vi "Simulation Acquired Data.vi"() -> ()   [LabVIEW 2013]
panel:
  in  "Data Queue":refnum<queue>
  in  "Skip Back Button":bool
  in  "FF Speed":dbl=2.0
  in  "Progress":dbl(slide)=0.002 scale=0.0..1435.0
  in  "Seek Forward Button":bool
  in  "Media Stop Button":bool
  in  "Play Button":bool
  in  "Tabs":enum32{"Config", "X", "Y", "Voltage"}(tab)
  in  "Reset Graphs":bool
  in  "TDMS File Name":string
  in  "TDMS Output Folder":path
  out "TDMS Path Result":path
  in  "View Data After?":bool
  out "X Position":cluster{"Y":dbl[], "Y":dbl[]}[](graph)
  out "Y Position":cluster{"Y":dbl[], "Y":dbl[]}[](graph)
  out "Tip Voltage":cluster{"Y":dbl[], "Y":dbl[]}[](graph)
  in  "Background Image":refnum<vi>
  in  "Inkscape File (.svg)":refnum<vi>
  in  "Run":refnum<vi>
  in  "Abort":refnum<vi>
  in  "Lithography Data":T1(array[cluster])
  # "Will be used for TDMS playback"
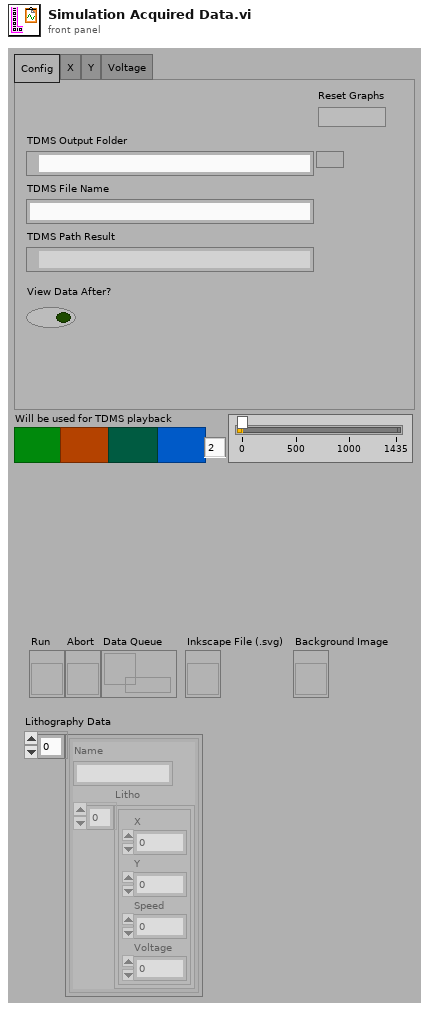
[diagram p1: front panel]
types:
  T1 = cluster{"Name":string, "Litho":cluster{"X":dbl, "Y":dbl, "Speed":dbl, "Voltage":dbl}[]}[]
  T2 = cluster{"X":dbl, "Y":dbl, "Speed":dbl, "Voltage":dbl}[]
  T3 = cluster{"X":dbl, "Y":dbl, "Speed":dbl, "Voltage":dbl}
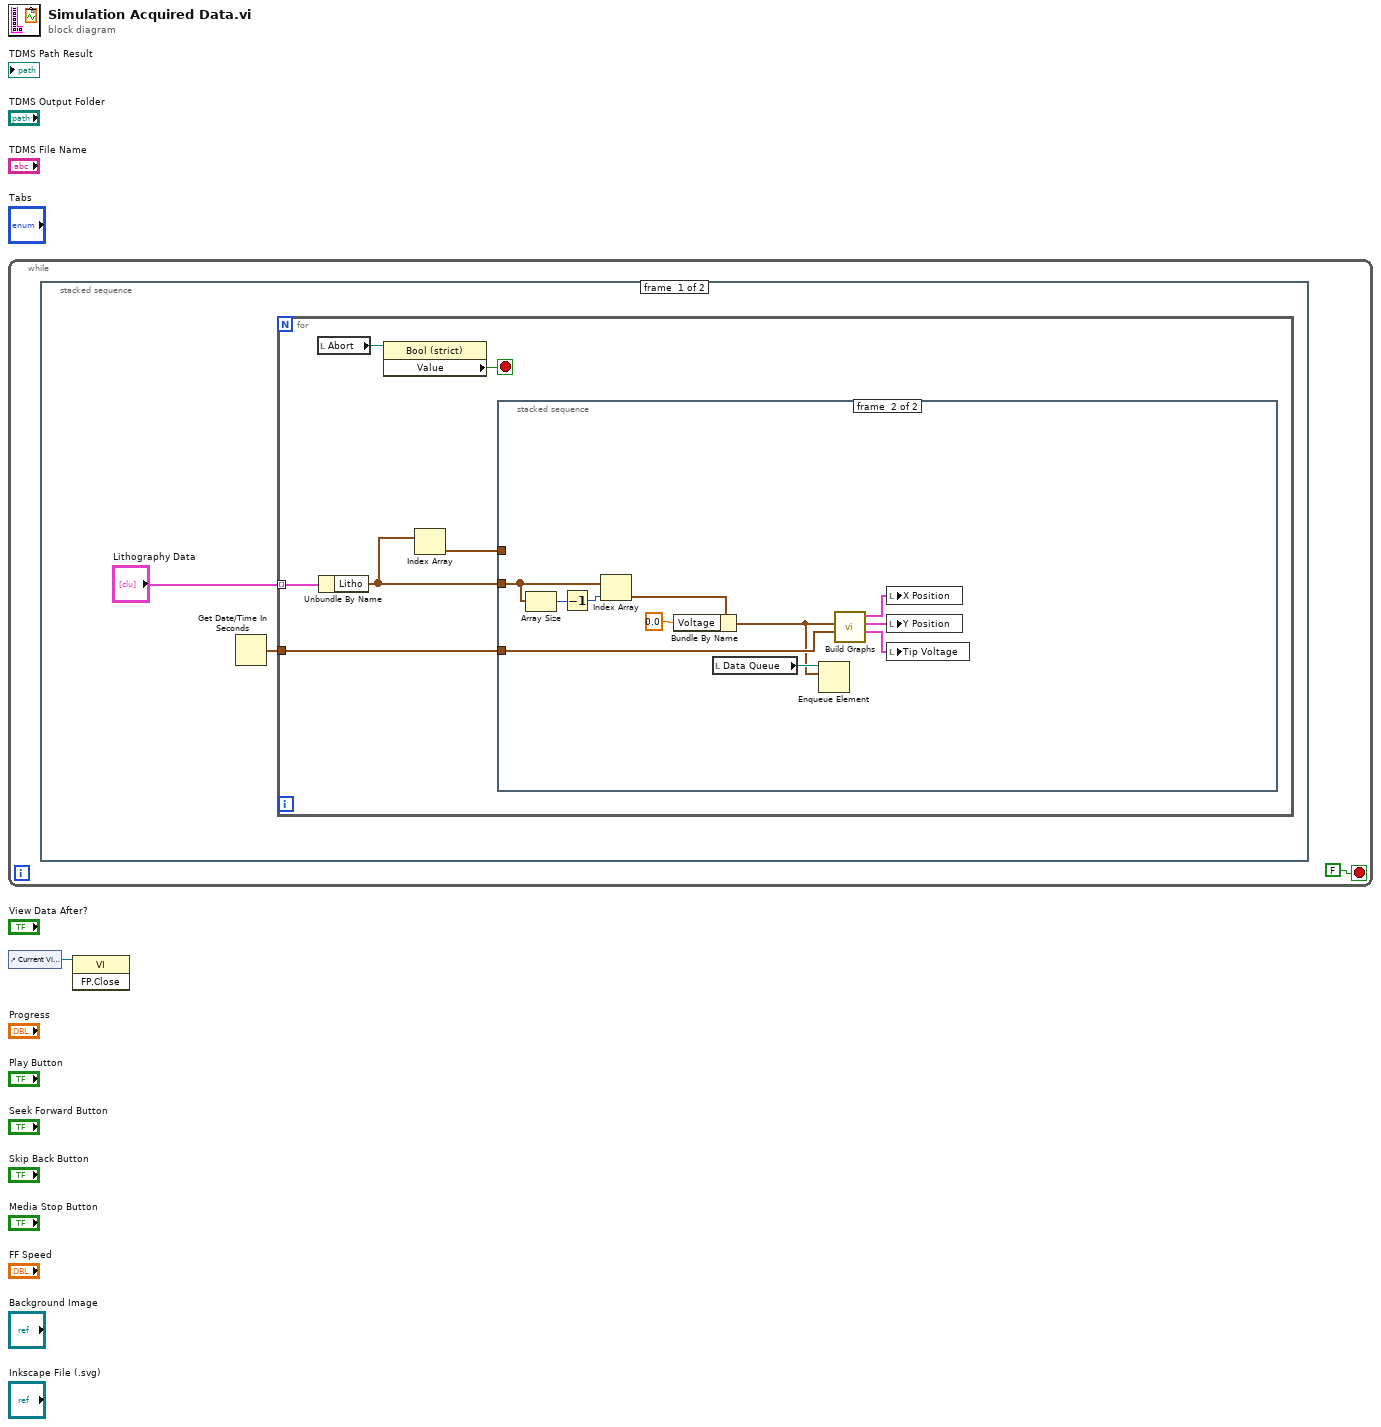
[diagram p0: block diagram]
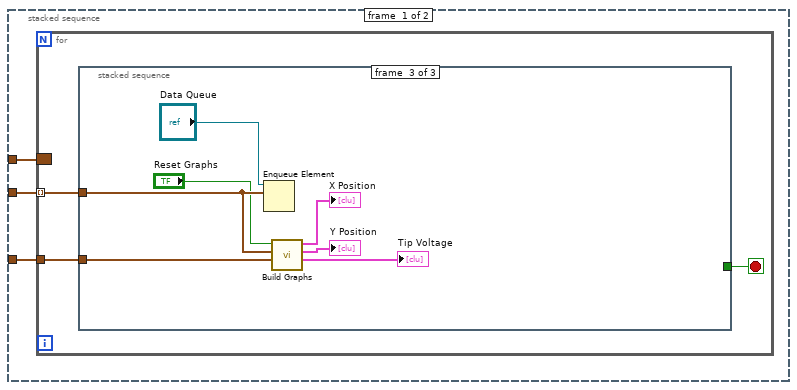
[diagram p2: hidden frame]
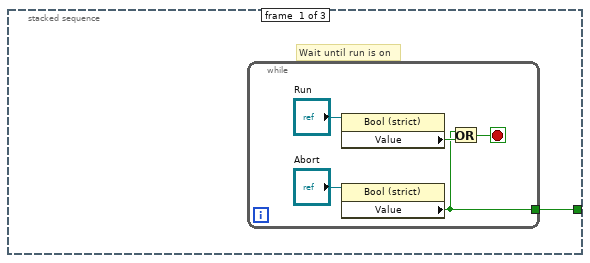
[diagram p3: hidden frame]
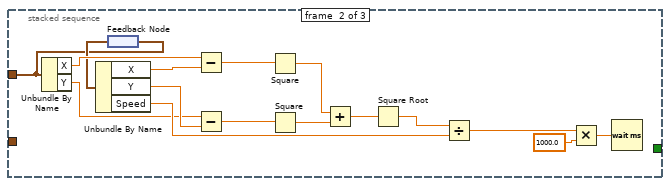
[diagram p4: hidden frame]
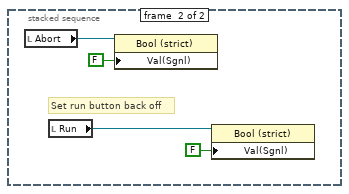
[diagram p5: hidden frame]
diagram:
  n1 = while {
    stop <- FALSE stop-if-true
    n2 = stacked-sequence {
      frame #0 {
        n3 = Get Date/Time In Seconds() -> (seconds since 1Jan1904=w3:timestamp)
        n4 = for {
          tunnel: "Lithography Data" -> [w10] mode=indexing
          tunnel: w3 -> [w5]
          stop <- w7 stop-if-true
          n5 = local read "Abort"() -> (w6:refnum<vi>)
          n6 = Unbundle By Name(w10) -> ("Litho"=w8:T2)
          n7 = property class="Bool (strict)"(reference=w6) -> ("Value"=w7:bool)  [unwired: 1 in, 2 out]
          n8 = Index Array(array=w8) -> (element=w9:T3)  [unwired: 1 in]
          n9 = stacked-sequence {
            tunnel: w9 -> [w13 _]
            tunnel: w8 -> [w12 w54]
            tunnel: w5 -> [w11 w51]
            frame #0 {
              n10 = for {
                tunnel: w12 -> [w16] mode=indexing
                border: w13 -> [_]
                tunnel: w11 -> [w14]
                stop <- w15 stop-if-true
                n11 = stacked-sequence {
                  tunnel: w16 -> [_ w23 w44]
                  tunnel: [w17 _ _] -> w15
                  tunnel: w14 -> [_ _ w43]
                  frame #0 {
                    # "Wait until run is on"
                    n12 = while {
                      tunnel: [w20] -> w17
                      stop <- w22 stop-if-true
                      n13 = property class="Bool (strict)"(reference="Run") -> ("Value"=w21:bool)  [unwired: 1 in, 2 out]
                      n14 = property class="Bool (strict)"(reference="Abort") -> ("Value"=w20:bool)  [unwired: 1 in, 2 out]
                      n15 = Or(x=w20, y=w21) -> (x .or. y?=w22:bool)
                    }
                  }
                  frame #1 {
                    n16 = Unbundle By Name(w23) -> ("X"=w32:dbl, "Y"=w35:dbl)
                    n17 = feedback #1() -> (w31:T3)
                    n18 = Unbundle By Name(w31) -> ("X"=w33:dbl, "Y"=w36:dbl, "Speed"=w38:dbl)
                    n19 = feedback-in #1(w23) -> ()
                    n20 = Subtract(x=w32, y=w33) -> (x-y=w34:dbl)
                    n21 = Subtract(x=w35, y=w36) -> (x-y=w37:dbl)
                    n22 = Square(x=w34) -> (x^2=w27:dbl)
                    n23 = Square(x=w37) -> (x^2=w28:dbl)
                    n24 = Add(x=w27, y=w28) -> (x+y=w29:dbl)
                    n25 = Square Root(x=w29) -> (sqrt(x)=w30:dbl)
                    n26 = Divide(x=w30, y=w38) -> (x/y=w25:dbl)
                    n27 = Multiply(x=w25, y=1000.0) -> (x*y=w26:dbl)
                    n28 = Wait (ms)(milliseconds to wait=w26) -> ()  [unwired: 1 out]
                  }
                  frame #2 {
                    n29 = Enqueue Element(queue="Data Queue", element=w44) -> ()  [unwired: 2 in, 3 out]
                    n30 = call "Build Graphs.vi"("Start Time in Seconds"=w43, "Litho Point"=w44, "Reset Graphs"="Reset Graphs") -> ("Voltage"=→"Tip Voltage":cluster{"X":dbl[], "Y":dbl[]}[], "Y Position"=→"Y Position":cluster{"X":dbl[], "Y":dbl[]}[], "X Position"=→"X Position":cluster{"X":dbl[], "Y":dbl[]}[])  [unwired: 6 in]
                  }
                }
              }
            }
            frame #1 {
              n31 = Array Size(array=w54) -> (size(s)=w56:i32)
              n32 = Decrement(x=w56) -> (x-1=w55:i32)
              n33 = Index Array(array=w54, index=w55) -> (element=w53:T3)
              n34 = Bundle By Name(cluster=w53, "Voltage"=0.0) -> (w46:T3)
              n35 = local read "Data Queue"() -> (w47:refnum<queue>)
              n36 = Enqueue Element(queue=w47, element=w46) -> ()  [unwired: 2 in, 3 out]
              n37 = call "Build Graphs.vi"("Start Time in Seconds"=w51, "Litho Point"=w46) -> ("Voltage"=w48:cluster{"X":dbl[], "Y":dbl[]}[], "Y Position"=w49:cluster{"X":dbl[], "Y":dbl[]}[], "X Position"=w50:cluster{"X":dbl[], "Y":dbl[]}[])  [unwired: 7 in]
              n38 = local write "X Position"(w50) -> ()
              n39 = local write "Y Position"(w49) -> ()
              n40 = local write "Tip Voltage"(w48) -> ()
            }
          }
        }
      }
      frame #1 {
        # "Set run button back off"
        n41 = local read "Abort"() -> (w58:refnum<vi>)
        n42 = local read "Run"() -> (w59:refnum<vi>)
        n43 = property class="Bool (strict)"(reference=w58, "Val(Sgnl)"=FALSE ("Value (Signaling)")) -> ()  [unwired: 1 in, 2 out]
        n44 = property class="Bool (strict)"(reference=w59, "Val(Sgnl)"=FALSE ("Value (Signaling)")) -> ()  [unwired: 1 in, 2 out]
      }
    }
  }
  n45 = control-ref of="Current VI Reference"() -> (w1:refnum<vi>)
  n46 = invoke class="VI" method="FP.Close"(reference=w1) -> ()  [unwired: 2 in, 3 out]
